vi "Convert Metadata to Temp.vi"(8 "error in (no error)":errorcluster, 10 "Temp Metadata":u16[](array[numeric]), 11 "Optris PI in":refnum<class "Optris PI.lvclass">) -> (0 "error out":errorcluster, 2 "Temperatures (Def. C)":dbl[](array[numeric]), 3 "Optris PI out":refnum<class "Optris PI.lvclass">)   [LabVIEW 2018, in "Optris PI.lvlib" / "Optris PI.lvclass"]
uses:
  Optris PI.lvclass
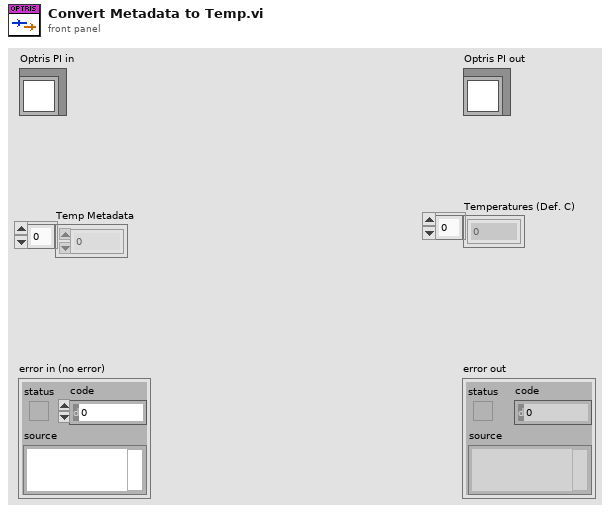
[diagram p1: front panel]
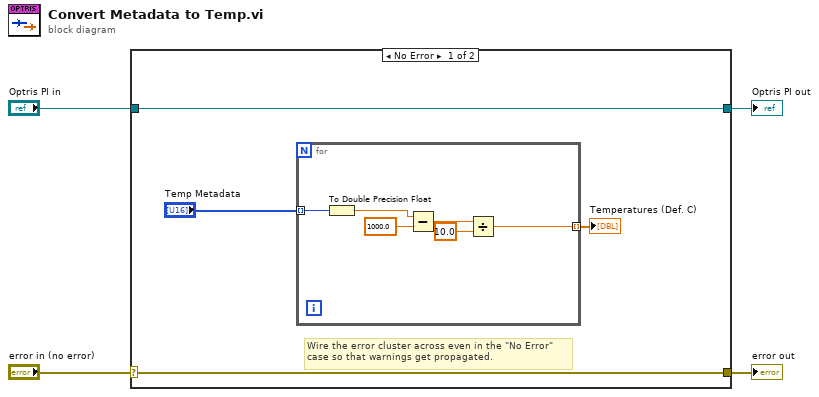
[diagram p0: block diagram]
diagram:
  n1 = case shown="No Error" "error in (no error)" {
    selector: "error in (no error)" -> [w7 w16]
    tunnel: [w7 w16] -> w3
    tunnel: [w8 w15] -> w1
    tunnel: "Optris PI in" -> [w8 w15]
    frame No Error {
      # "Wire the error cluster across even in the \"No Error\"\ncase so that warnings get propagated."
      n2 = for {
        tunnel: "Temp Metadata" -> [w14] mode=indexing
        tunnel: [w9] -> w5 mode=indexing
        n3 = To Double Precision Float(number=w14) -> (double precision float=w13:dbl)
        n4 = Subtract(x=w13, y=1000.0) -> (x-y=w11:dbl)
        n5 = Divide(x=w11, y=10.0) -> (x/y=w9:dbl)
      }
      "Temperatures (Def. C)" <- w5
    }
    frame Error {
    }
  }
  "error out" <- w3
  "Optris PI out" <- w1
